vi "JGPR3_TicTacToe.vi"() -> ()   [LabVIEW 2019]
doc: "TIc Tac Toe Vs Bot \n\nJuan Gamez\nP3600\nCSUSB Physics"
uses:
  typedefs/tic-tac-toe board.ctl
  typedefs/x or o or empty.ctl
  typedefs/invisible buttons.ctl
  typedefs/tic-tac-toe data.ctl
  typedefs/tic-tac-toe state enum.ctl
  typedefs/turn enum.ctl
  typedefs/game status.ctl
panel:
  out "o turn":bool=TRUE
  out "x turn":bool=TRUE
  in  "buttons":T1={"00"=TRUE, "01"=FALSE, "02"=FALSE, "10"=FALSE, "11"=FALSE, "12"=FALSE, "20"=FALSE, "21"=FALSE, "22"=FALSE}
  out "stalemate":bool=TRUE
  out "o wins":bool=TRUE
  out "x wins":bool=TRUE
  out "Game Board":T2
  # "Tic Tac Toe"
  # "Tic Tac Toe VS Super Hard A.I\nJuan Gamez\nP3600"
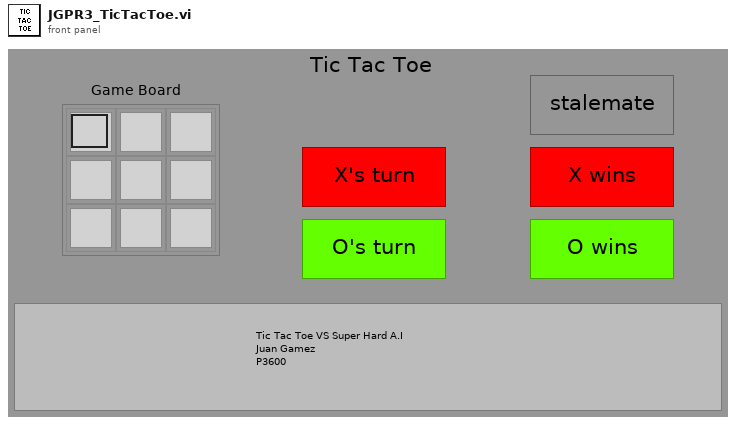
[diagram p1: front panel]
types:
  T1 = typedef "invisible buttons.ctl" = cluster{"00":bool, "01":bool, "02":bool, "10":bool, "11":bool, "12":bool, "20":bool, "21":bool, "22":bool}
  T2 = typedef "tic-tac-toe board.ctl" = T3[][]
  T3 = typedef "x or o or empty.ctl" = u16
  T4 = typedef "tic-tac-toe state enum.ctl" = enum16{"start game", "clear", "x turn", "o turn", "legal move", "update board", "evaluate board", "turn decide", "game over"}
  T5 = typedef "tic-tac-toe data.ctl" = cluster{"state":T4, "display board":u16[][], "eval board":i32[][], "turn":T6, "desired move":bool[][], "game status":T7}
  T6 = typedef "turn enum.ctl" = enum32{"x turn", "o turn"}
  T7 = typedef "game status.ctl" = enum16{"not over", "over stalemate", "over x wins", "over o wins"}
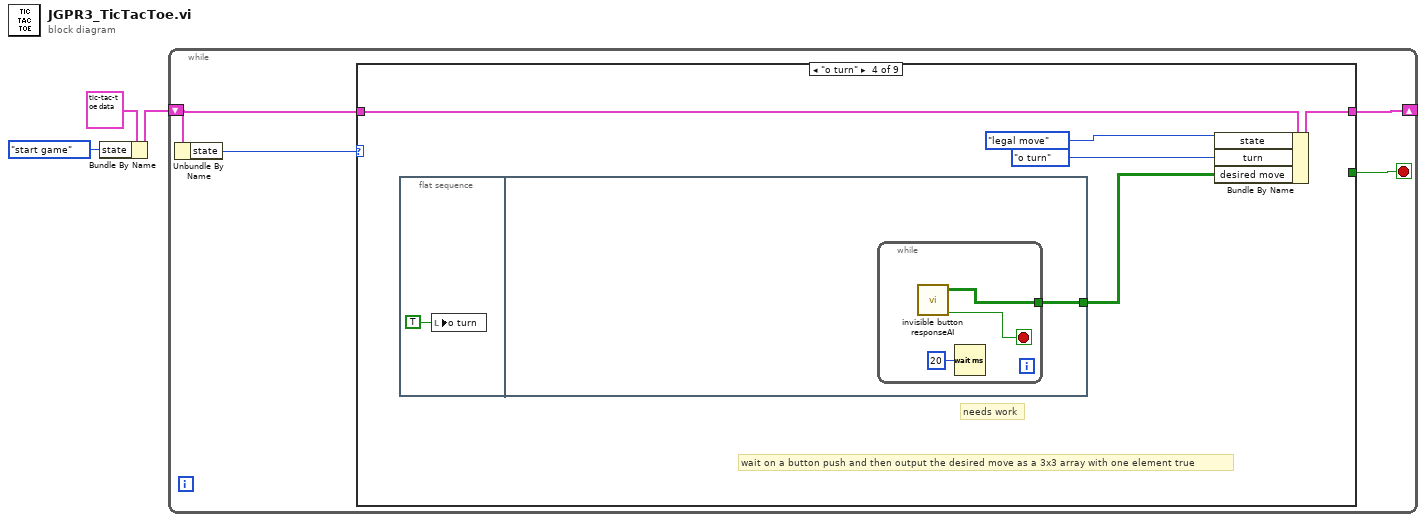
[diagram p0: block diagram]
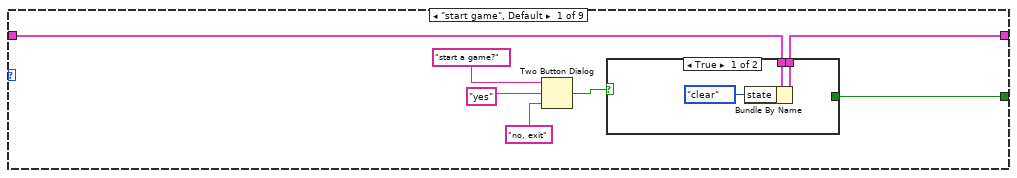
[diagram p2: hidden frame]
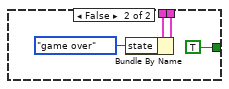
[diagram p3: hidden frame]
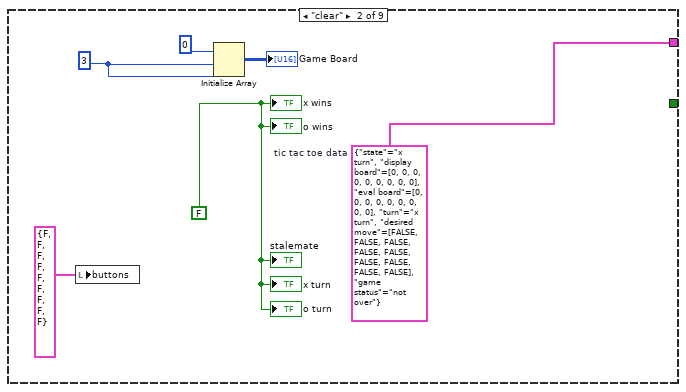
[diagram p4: hidden frame]
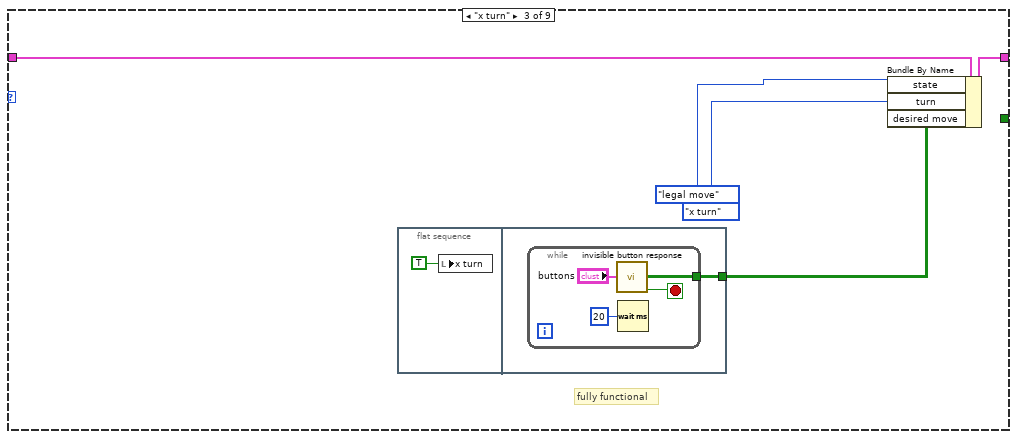
[diagram p5: hidden frame]
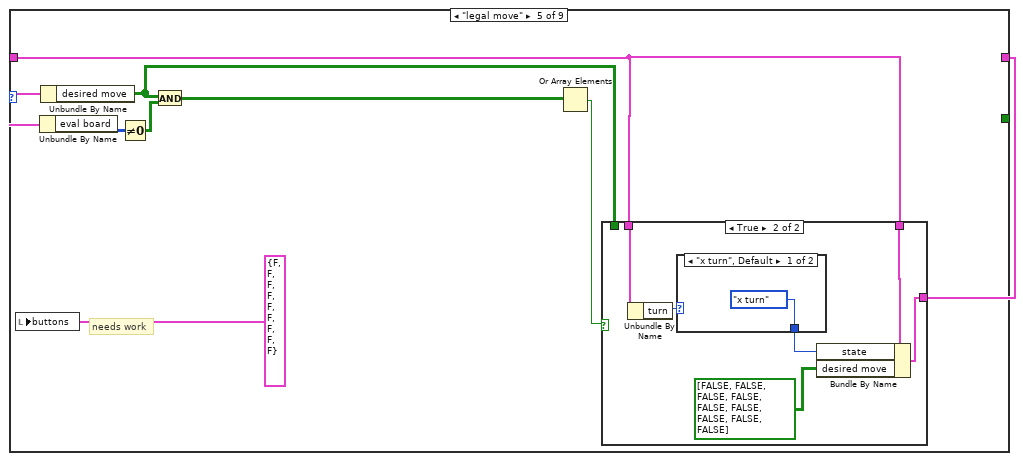
[diagram p6: hidden frame]
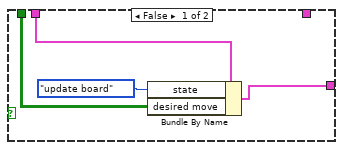
[diagram p7: hidden frame]
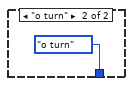
[diagram p8: hidden frame]
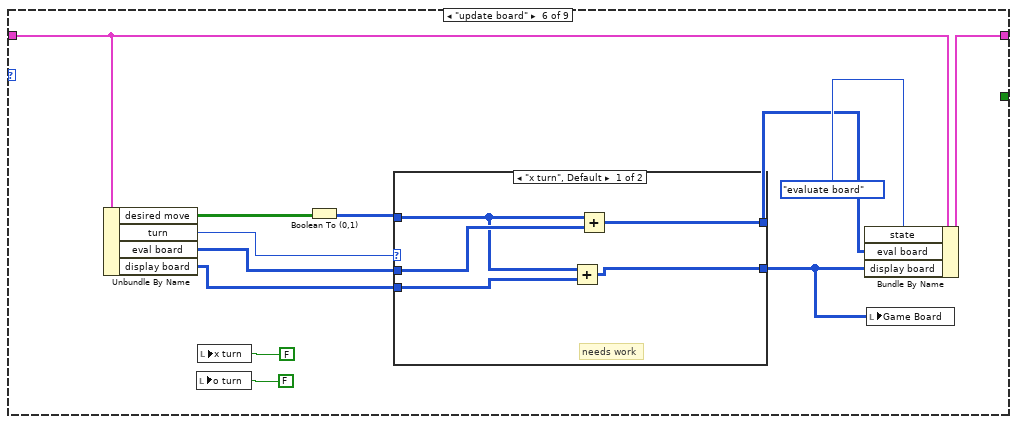
[diagram p9: hidden frame]
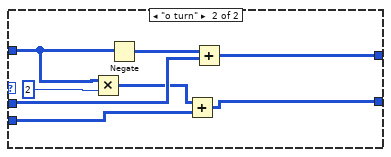
[diagram p10: hidden frame]
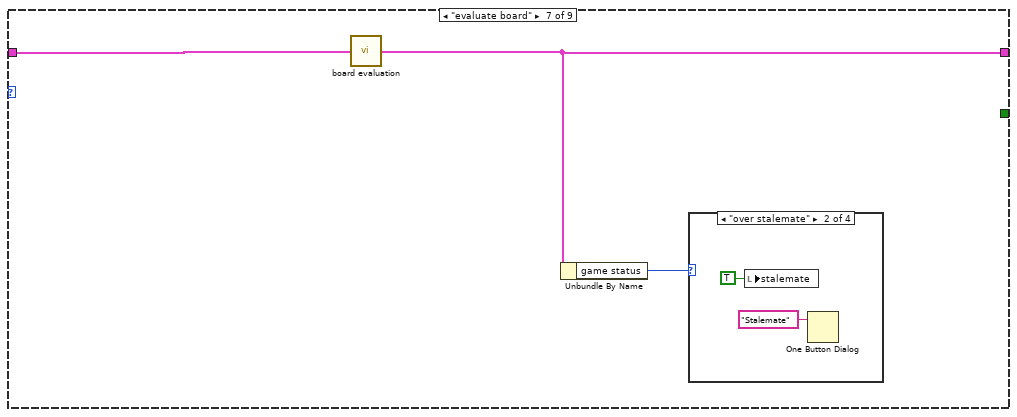
[diagram p11: hidden frame]
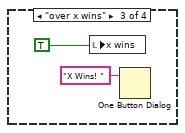
[diagram p13: hidden frame]
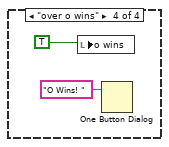
[diagram p14: hidden frame]
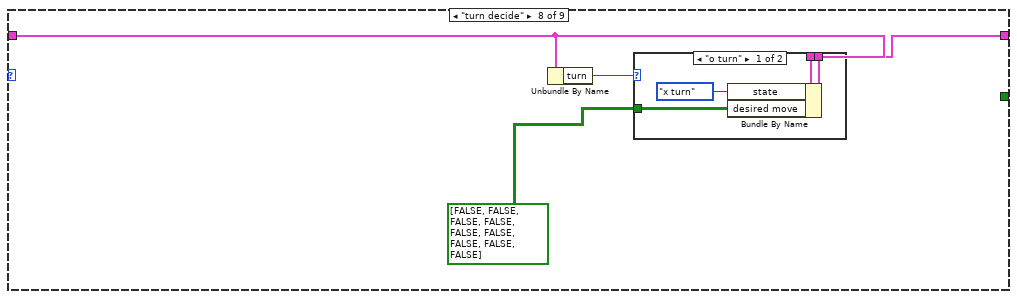
[diagram p15: hidden frame]
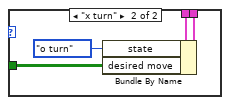
[diagram p16: hidden frame]
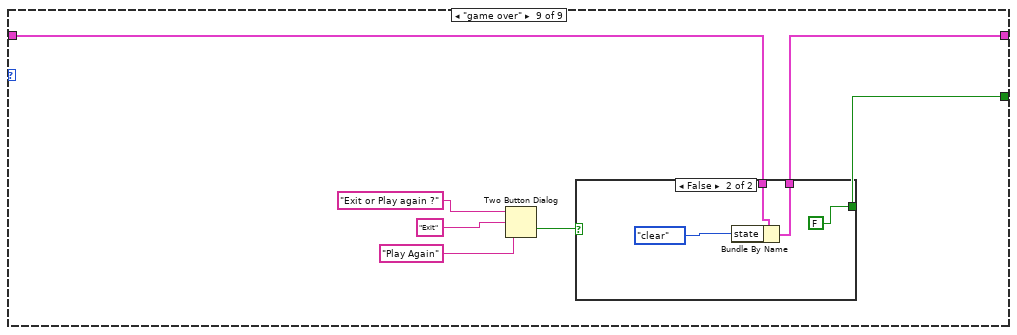
[diagram p17: hidden frame]
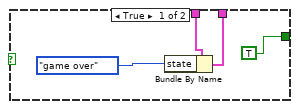
[diagram p18: hidden frame]
diagram:
  n1 = Bundle By Name(cluster=T5 {"state"=enum."start game", "display board"=[[0, 0, 0], [0, 0, 0], [0, 0, 0]], "eval board"=[[0, 0, 0], [0, 0, 0], [0, 0, 0]], "turn"=enum."x turn", "desired move"=[[FALSE, FALSE, FALSE], [FALSE, FALSE, FALSE], [FALSE, FALSE, FALSE]], "game status"=enum."not over"} ("tic tac toe data"), "state"=tic-tac-toe_state_enum."start game") -> (w2:T5)
  n2 = while {
    shift-right: [w5] -> _
    shift-left: w2 -> [w6]
    stop <- w4 stop-if-true
    n3 = Unbundle By Name(w6) -> ("state"=w7:T4)
    n4 = case shown="\"o turn\"" w7 {
      tunnel: w6 -> [w14 _ w30 w43 w51 w80 w95 w106 w117]
      tunnel: [w10 w27 w29 w42 w50 w71 w94 w105 w116] -> w5
      tunnel: [w8 _ _ _ _ _ _ _ w115] -> w4
      frame "start game", Default {
        n5 = Two Button Dialog(message="start a game?", 1:"no, exit" ("F button name (\"Cancel\")"), 2:"yes" ("T button name (\"OK\")")) -> (T button?=w9:bool)
        n6 = case shown="True" w9 {
          tunnel: w14 -> [w17 w21]
          tunnel: [w16 w20] -> w10
          tunnel: [_ TRUE] -> w8
          frame True {
            n7 = Bundle By Name(cluster=w17, "state"=tic-tac-toe_state_enum."clear") -> (w16:T5)
          }
          frame False {
            n8 = Bundle By Name(cluster=w21, "state"=tic-tac-toe_state_enum."game over") -> (w20:T5)
          }
        }
      }
      frame "clear" {
        w27 = T5 {"state"=enum."x turn", "display board"=[[0, 0, 0], [0, 0, 0], [0, 0, 0]], "eval board"=[[0, 0, 0], [0, 0, 0], [0, 0, 0]], "turn"=enum."x turn", "desired move"=[[FALSE, FALSE, FALSE], [FALSE, FALSE, FALSE], [FALSE, FALSE, FALSE]], "game status"=enum."not over"}  # tic tac toe data
        w22 = FALSE ("x wins")
        w25 = 3 ("dimension size")
        n9 = local write "buttons"(T1 {"00"=FALSE, "01"=FALSE, "02"=FALSE, "10"=FALSE, "11"=FALSE, "12"=FALSE, "20"=FALSE, "21"=FALSE, "22"=FALSE} ("buttons")) -> ()
        n10 = Initialize Array(u16 0, w25, w25) -> (→"Game Board":u16[][])
        "x wins" <- w22
        "o wins" <- w22
        "stalemate" <- w22
        "o turn" <- w22
        "x turn" <- w22
      }
      frame "x turn" {
        # "fully functional"
        n11 = flat-sequence {
          tunnel: [w34] -> w28
          frame #0 {
            n12 = local write "x turn"(TRUE ("x turn")) -> ()
          }
          frame #1 {
            n13 = while {
              tunnel: [w37] -> w34
              stop <- w36 stop-if-true
              n14 = call "invisible button response.vi"("invisible buttons"="buttons") -> ("desired move"=w37:bool[][], "stop loop"=w36:bool)  [unwired: 13 in]
              n15 = Wait (ms)(milliseconds to wait=u32 20) -> ()  [unwired: 1 out]
            }
          }
        }
        n16 = Bundle By Name(cluster=w30, "state"=tic-tac-toe_state_enum."legal move", "turn"=turn_enum."x turn", "desired move"=w28) -> (w29:T5)
      }
      frame "o turn" {
        # "wait on a button push and then output the desired move as a 3x3 array with one element true"
        # "needs work"
        n17 = flat-sequence {
          tunnel: [w45] -> w39
          frame #0 {
            n18 = local write "o turn"(TRUE ("x turn")) -> ()
          }
          frame #1 {
            n19 = while {
              tunnel: [w47] -> w45
              stop <- w46 stop-if-true
              n20 = call "invisible button responseAI.vi"() -> ("desired move"=w47:bool[][], "stop loop"=w46:bool)  [unwired: 14 in]
              n21 = Wait (ms)(milliseconds to wait=u32 20) -> ()  [unwired: 1 out]
            }
          }
        }
        n22 = Bundle By Name(cluster=w43, "state"=tic-tac-toe_state_enum."legal move", "turn"=turn_enum."o turn", "desired move"=w39) -> (w42:T5)
      }
      frame "legal move" {
        # "needs work"
        n23 = local write "buttons"(T1 {"00"=FALSE, "01"=FALSE, "02"=FALSE, "10"=FALSE, "11"=FALSE, "12"=FALSE, "20"=FALSE, "21"=FALSE, "22"=FALSE} ("buttons")) -> ()
        n24 = Unbundle By Name(w51) -> ("eval board"=w55:i32[][])
        n25 = Unbundle By Name(w51) -> ("desired move"=w49:bool[][])
        n26 = Not Equal To 0?(x=w55) -> (x != 0?=w54:bool[][])
        n27 = And(x=w49, y=w54) -> (x .and. y?=w53:bool[][])
        n28 = Or Array Elements(Boolean array=w53) -> (logical OR=w52:bool)
        n29 = case shown="True" w52 {
          tunnel: w51 -> [w59 w66]
          tunnel: w51 -> [_ w64]
          tunnel: [w57 w63] -> w50
          tunnel: w49 -> [w58 _]
          frame False {
            n30 = Bundle By Name(cluster=w59, "state"=tic-tac-toe_state_enum."update board", "desired move"=w58) -> (w57:T5)
          }
          frame True {
            n31 = Unbundle By Name(w66) -> ("turn"=w65:T6)
            n32 = case shown="\"x turn\", Default" w65 {
              tunnel: [tic-tac-toe_state_enum."x turn" ("state") tic-tac-toe_state_enum."o turn" ("state")] -> w62
              frame "x turn", Default {
              }
              frame "o turn" {
              }
            }
            n33 = Bundle By Name(cluster=w64, "state"=w62, "desired move"=bool[][] [[FALSE, FALSE, FALSE], [FALSE, FALSE, FALSE], [FALSE, FALSE, FALSE]]) -> (w63:T5)
          }
        }
      }
      frame "update board" {
        n34 = Unbundle By Name(w80) -> ("desired move"=w76:bool[][], "turn"=w79:T6, "eval board"=w74:i32[][], "display board"=w73:u16[][])
        n35 = local write "o turn"(FALSE ("o turn")) -> ()
        n36 = local write "x turn"(FALSE ("x turn")) -> ()
        n37 = Boolean To (0,1)(Boolean=w76) -> (0, 1=w75:i16[][])
        n38 = case shown="\"x turn\", Default" w79 {
          tunnel: w75 -> [w83 w87]
          tunnel: w74 -> [w85 w93]
          tunnel: w73 -> [w84 w92]
          tunnel: [w82 w91] -> w70
          tunnel: [w81 w90] -> w69
          frame "x turn", Default {
            # "needs work"
            n39 = Add(x=w83, y=w84) -> (x+y=w82:u16[][])
            n40 = Add(x=w83, y=w85) -> (x+y=w81:i32[][])
          }
          frame "o turn" {
            n41 = Multiply(x=w87, y=2) -> (x*y=w88:i32[][])
            n42 = Negate(x=w87) -> (-x=w86:i16[][])
            n43 = Add(x=w88, y=w92) -> (x+y=w91:i32[][])
            n44 = Add(x=w86, y=w93) -> (x+y=w90:i32[][])
          }
        }
        n45 = Bundle By Name(cluster=w80, "state"=tic-tac-toe_state_enum."evaluate board", "eval board"=w69, "display board"=w70) -> (w71:T5)
        n46 = local write "Game Board"(w70) -> ()
      }
      frame "evaluate board" {
        n47 = call "board evaluation.vi"("tic tac toe data in"=w95) -> ("tic tac toe data out"=w94:T5)  [unwired: 14 in]
        n48 = Unbundle By Name(w94) -> ("game status"=w96:T7)
        n49 = case shown="\"over stalemate\"" w96 {
          frame "not over" {
          }
          frame "over stalemate" {
            n50 = local write "stalemate"(TRUE ("stalemate")) -> ()
            n51 = One Button Dialog(message="Stalemate") -> ()  [unwired: 1 in, 1 out]
          }
          frame "over x wins" {
            n52 = local write "x wins"(TRUE ("stalemate")) -> ()
            n53 = One Button Dialog(message="X Wins! ") -> ()  [unwired: 1 in, 1 out]
          }
          frame "over o wins" {
            n54 = local write "o wins"(TRUE ("stalemate")) -> ()
            n55 = One Button Dialog(message="O Wins! ") -> ()  [unwired: 1 in, 1 out]
          }
        }
      }
      frame "turn decide" {
        n56 = Unbundle By Name(w106) -> ("turn"=w104:T6)
        n57 = case shown="\"o turn\"" w104 {
          tunnel: w106 -> [w110 w114]
          tunnel: [w109 w113] -> w105
          tunnel: bool[][] [[FALSE, FALSE, FALSE], [FALSE, FALSE, FALSE], [FALSE, FALSE, FALSE]] ("desired move") -> [w107 w111]
          frame "o turn" {
            n58 = Bundle By Name(cluster=w110, "state"=tic-tac-toe_state_enum."x turn", "desired move"=w107) -> (w109:T5)
          }
          frame "x turn" {
            n59 = Bundle By Name(cluster=w114, "state"=tic-tac-toe_state_enum."o turn", "desired move"=w111) -> (w113:T5)
          }
        }
      }
      frame "game over" {
        n60 = Two Button Dialog(message="Exit or Play again ?", 1:"Play Again" ("F button name (\"Cancel\")"), 2:"Exit" ("T button name (\"OK\")")) -> (T button?=w118:bool)
        n61 = case shown="False" w118 {
          tunnel: w117 -> [w124 w128]
          tunnel: [w123 w127] -> w116
          tunnel: [TRUE FALSE] -> w115
          frame True {
            n62 = Bundle By Name(cluster=w124, "state"=tic-tac-toe_state_enum."game over") -> (w123:T5)
          }
          frame False {
            n63 = Bundle By Name(cluster=w128, "state"=tic-tac-toe_state_enum."clear") -> (w127:T5)
          }
        }
      }
    }
  }
